vi "Do.vi"(8 "error in (no error)":errorcluster, 10 "Actor in":refnum<class "Actor.lvclass">, 11 "Initialize DLS Laser Msg in":refnum<class "Initialize FLS Laser Msg.lvclass">) -> (0 "error out":errorcluster, 2 "Actor out":refnum<class "Actor.lvclass">)   [LabVIEW 2018, in "FLS Laser Actor.lvlib" / "Initialize FLS Laser Msg.lvclass"]
uses:
  Initialize FLS Laser Msg.lvclass
  <vilib>/ActorFramework/Actor/Actor.lvclass
  FLS Laser Actor.lvclass
  C:/Program Files (x86)/National Instruments/LabVIEW 2018/vi.lib/ActorFramework/Actor/Actor.lvclass
  Initialize FLS Laser Msg.lvclass/Initialize FLS Laser Msg.ctl
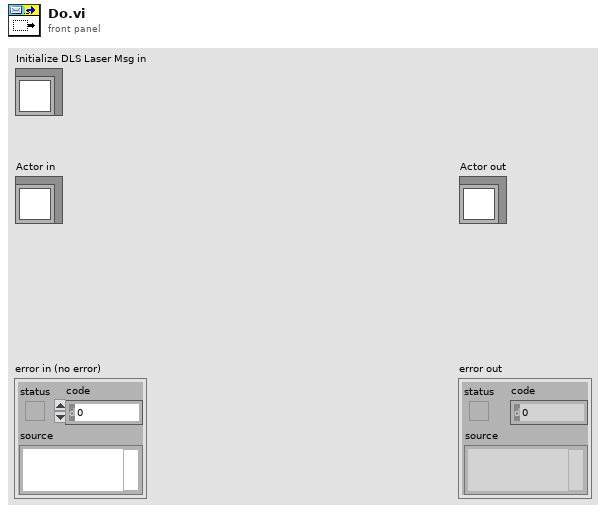
[diagram p1: front panel]
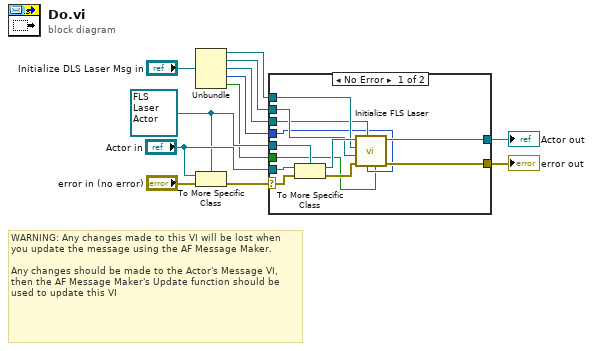
[diagram p0: block diagram]
diagram:
  w7 = refnum<class "FLS Laser Actor.lvclass"> refnum ("Actor Type")
  # "WARNING: Any changes made to this VI will be lost when you update the message using the AF Message Maker.\n\nAny changes should be made to the Actor's Message VI, then the AF Message Maker's Update function should be used to update this VI"
  n1 = Unbundle("Initialize DLS Laser Msg in") -> (w6:refnum<visa-resource-name>, w5:refnum<vi>, w4:refnum<vi>, w3:enum16{"A", "B", "C", "D"}, w2:bool)
  n2 = To More Specific Class(target class=w7, reference="Actor in", error in="error in (no error)") -> (error out=w11:errorcluster)  [unwired: 1 out]
  n3 = case shown="No Error" w11 {
    selector: w11 -> [w24 w26]
    tunnel: [w19 w26] -> w10
    tunnel: [w18 w25] -> w9
    tunnel: "Actor in" -> [w23 w25]
    tunnel: w7 -> [w22 _]
    tunnel: w6 -> [w17 _]
    tunnel: w5 -> [w16 _]
    tunnel: w4 -> [w15 _]
    tunnel: w3 -> [w14 _]
    tunnel: w2 -> [w13 _]
    frame No Error {
      n4 = To More Specific Class ("Actor Cast")(target class=w22, reference=w23, error in=w24) -> (specific class reference=w21:refnum<class "FLS Laser Actor.lvclass">, error out=w20:errorcluster)
      n5 = call "Initialize FLS Laser.vi"("Fault?"=w13, "FLS Laser ID (A,B,C or D)"=w14, "FLS Status LEDs Refnum"=w15, "error in (no error)"=w20, "FLS Range Refnum"=w16, "FLS COM Port"=w17, "FLS Laser Actor in"=w21) -> ("error out"=w19:errorcluster, "DLS Laser Actor out"=w18:refnum<class "FLS Laser Actor.lvclass">)  [unwired: 3 in]
    }
    frame Error {
    }
  }
  "error out" <- w10
  "Actor out" <- w9
